vi "Write Baud Rate.vi"(8 "error in (no error)":errorcluster, 10 "Baud Rate":u32=9600, 11 "Serial Slave in":refnum<class "Serial Slave.lvclass">) -> (0 "error out":errorcluster, 3 "Serial Slave out":refnum<class "Serial Slave.lvclass">)   [LabVIEW 2021, in "Serial Slave.lvclass"]
uses:
  Serial Slave.lvclass
  Serial Slave.lvclass/Serial Slave.ctl
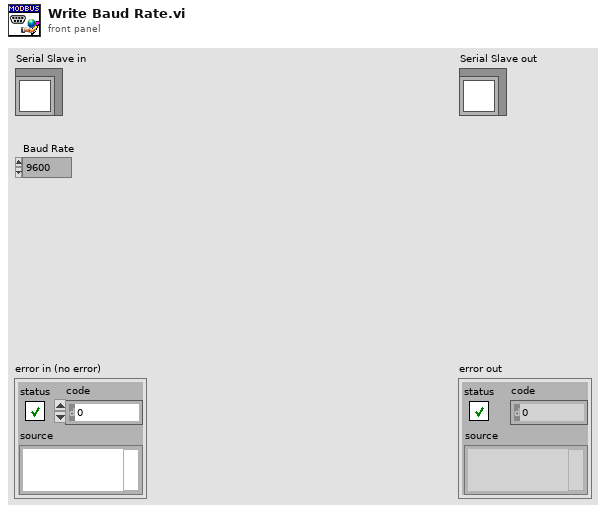
[diagram p1: front panel]
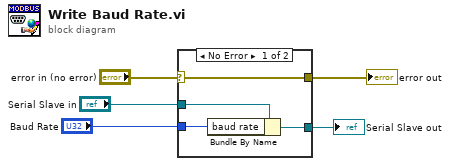
[diagram p0: block diagram]
diagram:
  n1 = case shown="No Error" "error in (no error)" {
    selector: "error in (no error)" -> [w9 w10]
    tunnel: [w9 w10] -> w4
    tunnel: [w7 w11] -> w2
    tunnel: "Serial Slave in" -> [w8 w11]
    tunnel: "Baud Rate" -> [w6 _]
    frame No Error {
      n2 = Bundle By Name(cluster=w8, "baud rate"=w6) -> (w7:refnum<class "Serial Slave.lvclass">)
    }
    frame Error {
    }
  }
  "error out" <- w4
  "Serial Slave out" <- w2
